vi "Get Buffer Size.vi"(0 "VISA resource name":refnum<visa-resource-name>, 5 "Buffer Name (defbuffer1)":string="defbuffer1", 11 "error in (no error)":errorcluster) -> (4 "VISA resource name out":refnum<visa-resource-name>, 6 "Buffer Size":i32, 15 "error out":errorcluster)   [LabVIEW 2021, in "Keithley 2450.lvlib"]
doc: "This indicates the number of readings a buffer can store."
uses:
  <instrlib>/Keithley 2450/Keithley 2450.lvlib
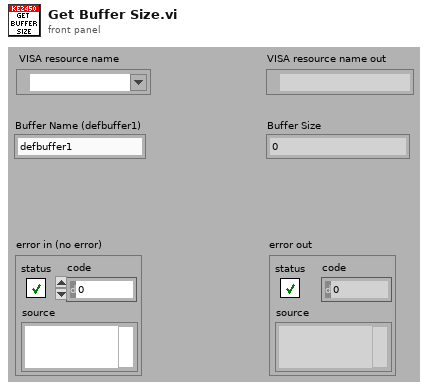
[diagram p1: front panel]
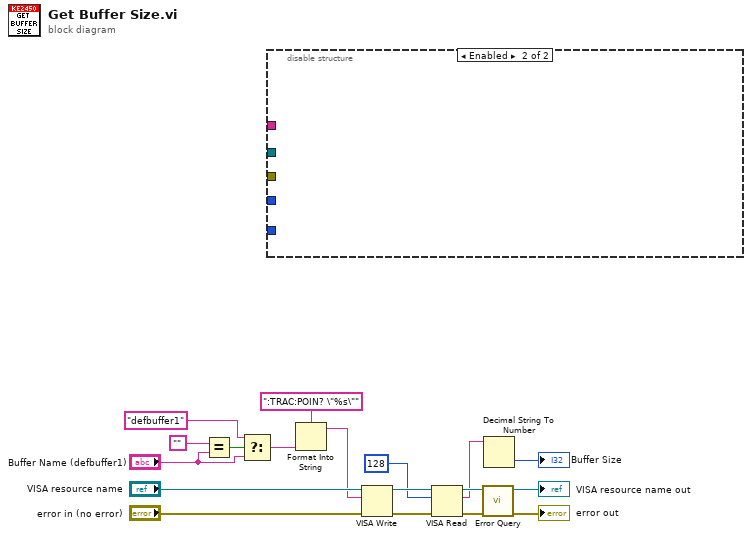
[diagram p0: block diagram]
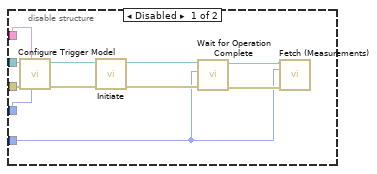
[diagram p2: hidden frame]
diagram:
  n1 = Equal?(x="", y="Buffer Name (defbuffer1)") -> (x = y?=w15:bool)
  n2 = Select(t="defbuffer1", s=w15, f="Buffer Name (defbuffer1)") -> (s? t:f=w8:string)
  n3 = disable-structure shown="Enabled" {
    disable-tunnel: _ -> [w25 _]
    disable-tunnel: _ -> [w24 _]
    disable-tunnel: _ -> [w23 _]
    disable-tunnel: _ -> [w22 _]
    disable-tunnel: _ -> [w19 _]
    frame Disabled {
      n4 = call <instrlib>:"Configure Trigger Model.vi"("Trigger Count (1)"=w24, "Buffer Name (defbuffer1)"=w19, "error in (no error)"=w22, "VISA resource name"=w23) -> ("error out"=w20:errorcluster, "VISA resource name out"=w21:refnum<visa-resource-name>)  [unwired: 6 in]
      n5 = call <instrlib>:"Initiate.vi"("error in (no error)"=w20, "VISA resource name"=w21) -> ("error out"=w28:errorcluster, "VISA resource name out"=w29:refnum<visa-resource-name>)  [unwired: 8 out]
      n6 = call <instrlib>:"Wait for Operation Complete.vi"("error in (no error)"=w28, "Timeout (10000 ms)"=w25, "VISA resource name"=w29) -> ("error out"=w27:errorcluster, "VISA resource name out"=w26:refnum<visa-resource-name>)  [unwired: 7 out]
      n7 = call <instrlib>:"Fetch (Measurements).vi"("VISA resource name"=w26, "Timeout (10000 ms)"=w25, "error in (no error)"=w27) -> ()  [unwired: 2 in, 11 out]
    }
    frame Enabled {
    }
  }
  n8 = Format Into String(format string=":TRAC:POIN? \"%s\"" ("Fetch Measurement"), w8) -> (resulting string=w9:string)  [unwired: 2 in, 1 out]
  n9 = VISA Write(VISA resource name="VISA resource name", write buffer=w9, error in (no error)="error in (no error)") -> (VISA resource name out=w7:refnum<visa-resource-name>, error out=w5:errorcluster)  [unwired: 1 out]
  n10 = VISA Read(VISA resource name=w7, byte count=u32 128, error in (no error)=w5) -> (VISA resource name out=w6:refnum<visa-resource-name>, read buffer=w2:string, error out=w4:errorcluster)  [unwired: 1 out]
  n11 = call <instrlib>:"Error Query.vi"("error in (no error)"=w4, "VISA resource name"=w6) -> ("error out"=→"error out":errorcluster, "VISA resource name out"=→"VISA resource name out":refnum<visa-resource-name>)  [unwired: 8 out]
  n12 = Decimal String To Number(string=w2) -> (number=→"Buffer Size":i32)  [unwired: 2 in, 1 out]
